vi "Power_to_string.vi"(11 "Horizontal Pointer Slide":dbl(slide) scale=0.0..100.0) -> (3 "Power string":string)   [LabVIEW 2020]
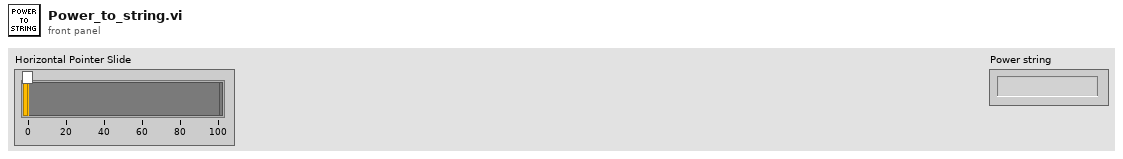
[diagram p1: front panel]
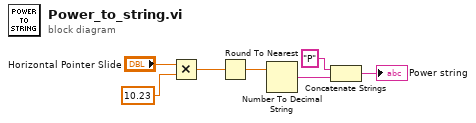
[diagram p0: block diagram]
diagram:
  n1 = Multiply(x="Horizontal Pointer Slide", y=10.23) -> (x*y=w5:dbl)
  n2 = Round To Nearest(number=w5) -> (nearest integer value=w4:dbl)
  n3 = Number To Decimal String(number=w4) -> (decimal integer string=w2:string)  [unwired: 1 in]
  n4 = Concatenate Strings("P" ("string"), w2) -> (→"Power string":string)
